vi "Close.vi"(8 "error in (no error)":errorcluster, 11 "Budgetizer in":refnum<class "Budgetizer.lvclass">) -> (0 "error out":errorcluster)   [LabVIEW 2018, in "Budgetizer.lvclass"]
uses:
  Budgetizer.lvclass
  Budgetizer.lvclass/Budgetizer.ctl
  database/Database.lvclass
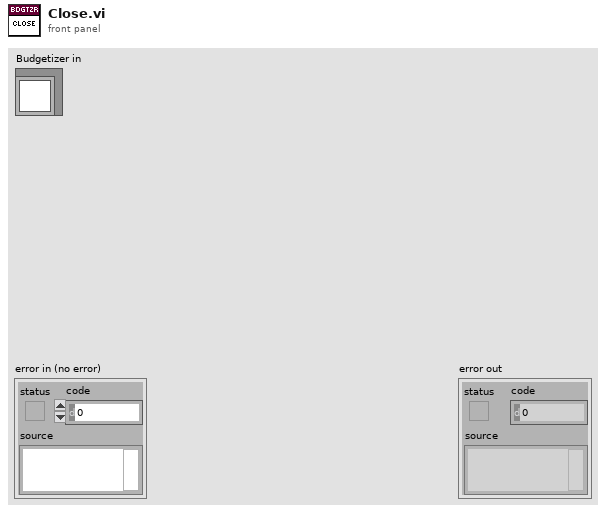
[diagram p1: front panel]
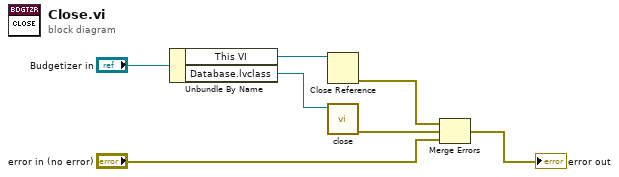
[diagram p0: block diagram]
diagram:
  n1 = Unbundle By Name("Budgetizer in") -> ("This VI"=w5:refnum<vi>, "Database.lvclass"=w6:refnum<class "Database.lvclass">)
  n2 = Close Reference(reference=w5) -> (error out=w4:errorcluster)  [unwired: 1 in]
  n3 = call "close.vi"("Database.lvclass"=w6) -> ("error out"=w3:errorcluster)  [unwired: 10 in]
  n4 = Merge Errors(w4, w3, "error in (no error)") -> (→"error out":errorcluster)
